vi "Random Temperature Noise.vi"() -> (0 "Temperature":dbl)   [LabVIEW 2013]
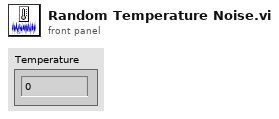
[diagram p1: front panel]
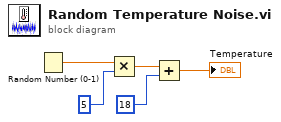
[diagram p0: block diagram]
diagram:
  n1 = Random Number (0-1)() -> (number: 0 to 1=w5:dbl)
  n2 = Multiply(x=w5, y=5) -> (x*y=w3:dbl)
  n3 = Add(x=w3, y=18) -> (x+y=→"Temperature":dbl)
